vi "CheckApplication.vi"(8 "error in (no error)":errorcluster, 11 "Application":string="YorkTownLight.exe") -> (0 "error out":errorcluster, 3 "Running?":bool)   [LabVIEW 2012]
panel:
  # "Type application name incl. extension\n\nWarning: CASE SENSITIVE\n\ne.g. YorkTownLight.exe"
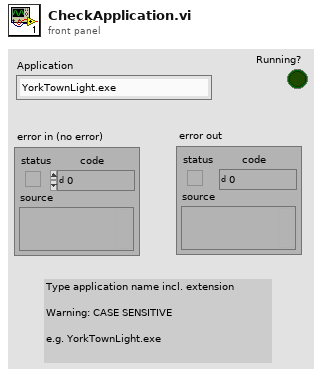
[diagram p1: front panel]
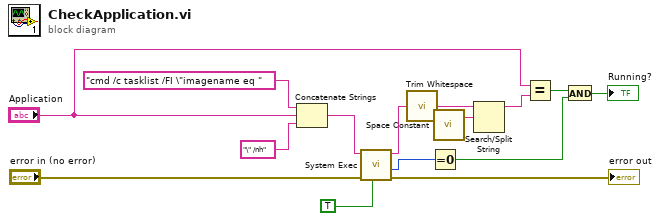
[diagram p0: block diagram]
diagram:
  n1 = Concatenate Strings("cmd /c tasklist /FI \"imagename eq " ("string"), "Application", "\" /nh" ("string")) -> (w10:string)
  n2 = call <vilib>:"System Exec.vi"("run minimized? (F)"=TRUE, "error in (no error)"="error in (no error)", "command line"=w10) -> ("error out"=→"error out":errorcluster, "return code"=w8:i32, "standard output"=w2:string)  [unwired: 5 in, 1 out]
  n3 = call <vilib>:"Trim Whitespace.vi"("string"=w2) -> ("trimmed string"=w1:string)  [unwired: 1 in]
  n4 = Equal To 0?(x=w8) -> (x = 0?=w5:bool)
  n5 = call <vilib>:"Space Constant.vi"() -> ("String"=w3:string)
  n6 = Search/Split String(string=w1, search string/char (-)=w3) -> (substring before match=w4:string)  [unwired: 1 in, 2 out]
  n7 = Equal?(x="Application", y=w4) -> (x = y?=w7:bool)
  n8 = And(x=w7, y=w5) -> (x .and. y?=→"Running?":bool)
